vi "Test.vi"() -> ()   [LabVIEW 2014, in "Generic Power Analyzer.lvlib" / "Tektronix PA1000.lvlib" / "Tektronix PA1000.lvclass"]
uses:
  Tektronix PA1000.lvclass
  <instrlib>/Tektronix PA1000/Tektronix PA1000.lvlib
panel:
  out "Foreground Data":dbl[](array[numeric])
  out "Displayed Number":i32
  out "Measurements Number":i32
  in  "VISA resource name":refnum<visa-resource-name>
  out "Measurement List":string[](array[string])
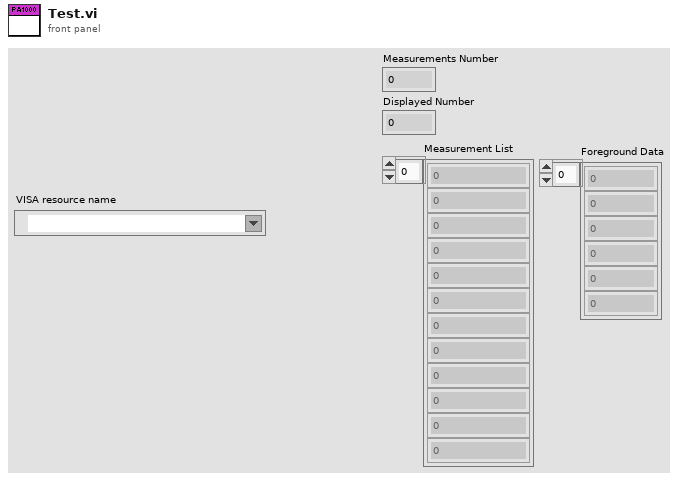
[diagram p1: front panel]
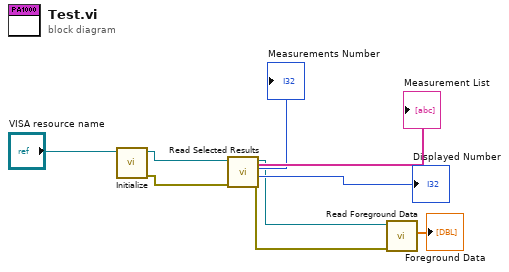
[diagram p0: block diagram]
diagram:
  n1 = call <instrlib>:"Initialize.vi"("VISA resource name"="VISA resource name") -> ("error out"=w8:errorcluster, "VISA resource name out"=w9:refnum<visa-resource-name>)  [unwired: 9 in]
  n2 = call <instrlib>:"Read Selected Results.vi"("error in (no error)"=w8, "VISA resource name"=w9) -> ("error out"=w2:errorcluster, "Displayed Number"=→"Displayed Number":i32, "Measurements Number"=→"Measurements Number":i32, "VISA resource name out"=w3:refnum<visa-resource-name>, "Measurement List"=→"Measurement List":string[])  [unwired: 5 in]
  n3 = call <instrlib>:"Read Foreground Data.vi"("error in (no error)"=w2, "VISA resource name"=w3) -> ("Foreground Data"=→"Foreground Data":dbl[])  [unwired: 7 in, 2 out]
